vi "Filter_Table_Test.vi"() -> ()   [LabVIEW 2025, in "Table_Filtering.lvlib"]
uses:
  Table_Filtering.lvlib
  <vilib>/Utility/miscctls.llb/LVRowAndColumnUnsignedTypeDef.ctl
panel:
  out "Error Out":errorcluster
  in  "Filter String":string="Protocol == UDP AND Length > 0.7 OR Source == 192.168.1.1 AND Hex_Data < 20"
  in  "Sort by":u16(ring) items=["Packet_Number", "Timestamp", "Source", "Destination", "Protocol", "Length", "Data", "Hex_Data"]
  in  "Headers and Types":string[][](array[string])=[["Packet_Number", "Timestamp", "Source", "Destination", "Protocol", "Length", "Data", "Hex_Data"], ["NUM", "STR", "STR", "STR", "STR", "NUM", "STR", "HEX"]]
  in  "Pause":bool
  out "Table Control":string[][](table)
  in  "stop":bool
  in  "Visible Columns":bool[](array[boolean])=[TRUE, TRUE, TRUE, TRUE, TRUE, TRUE, TRUE, TRUE]
  # "The filter expression uses the following syntax:\n\nSets of three arguments separated by logical operators.\nSpaces are used to separate keywords.\nEach set of three arguments follows the pattern: Field, Operator, Value.\nExample: \nProtocol == UDP AND Length > 0.7 OR Source == 192.168.1.1\n\nInvalid inputs include:\n\nStandalone logical operators (e.g., AND, OR)\nTerms by themselves\nArgument sets not equal to three in length\nParentheses\nIf an invalid filter is entered, a warning will be generated."
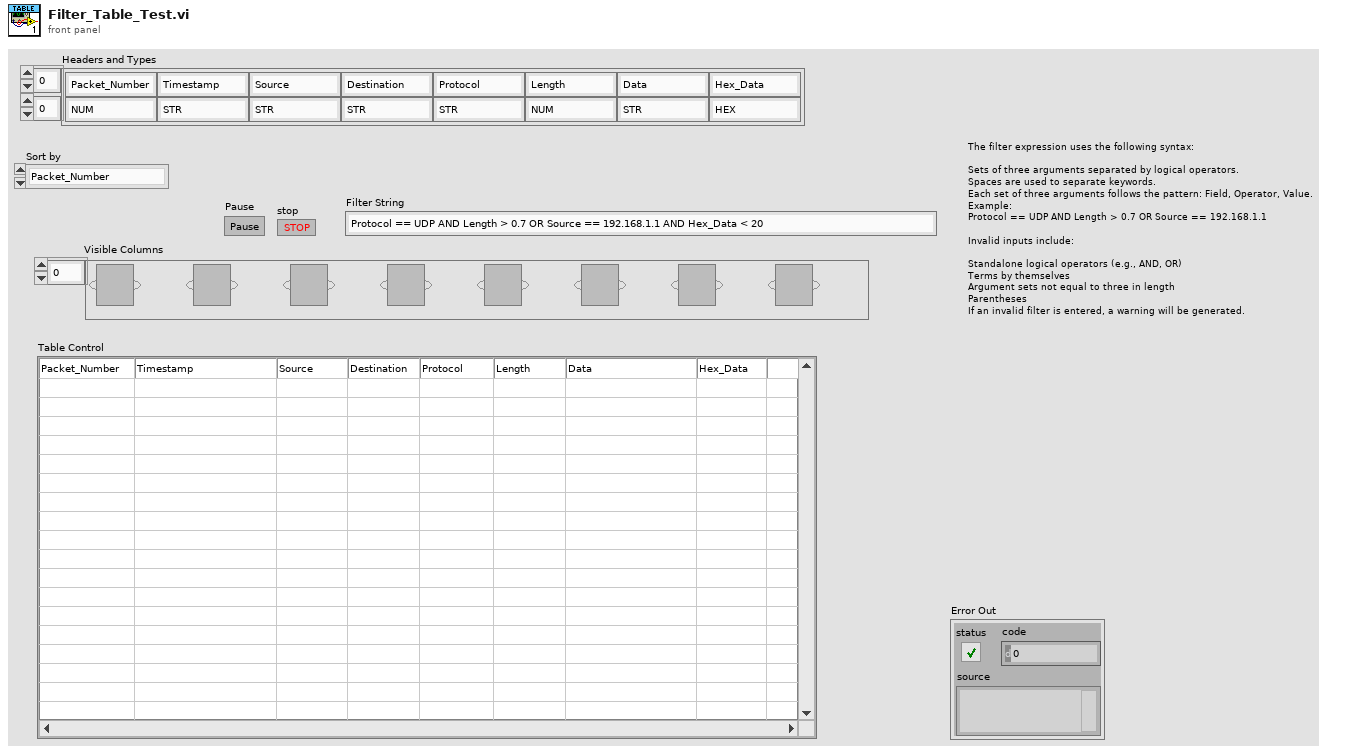
[diagram p1: front panel]
types:
  T1 = typedef "LVRowAndColumnUnsignedTypeDef.ctl" = cluster{"Row":u32, "Column":u32}
  T2 = cluster{"FIELD":string, "OPERATOR":string, "VALUE":string}[]
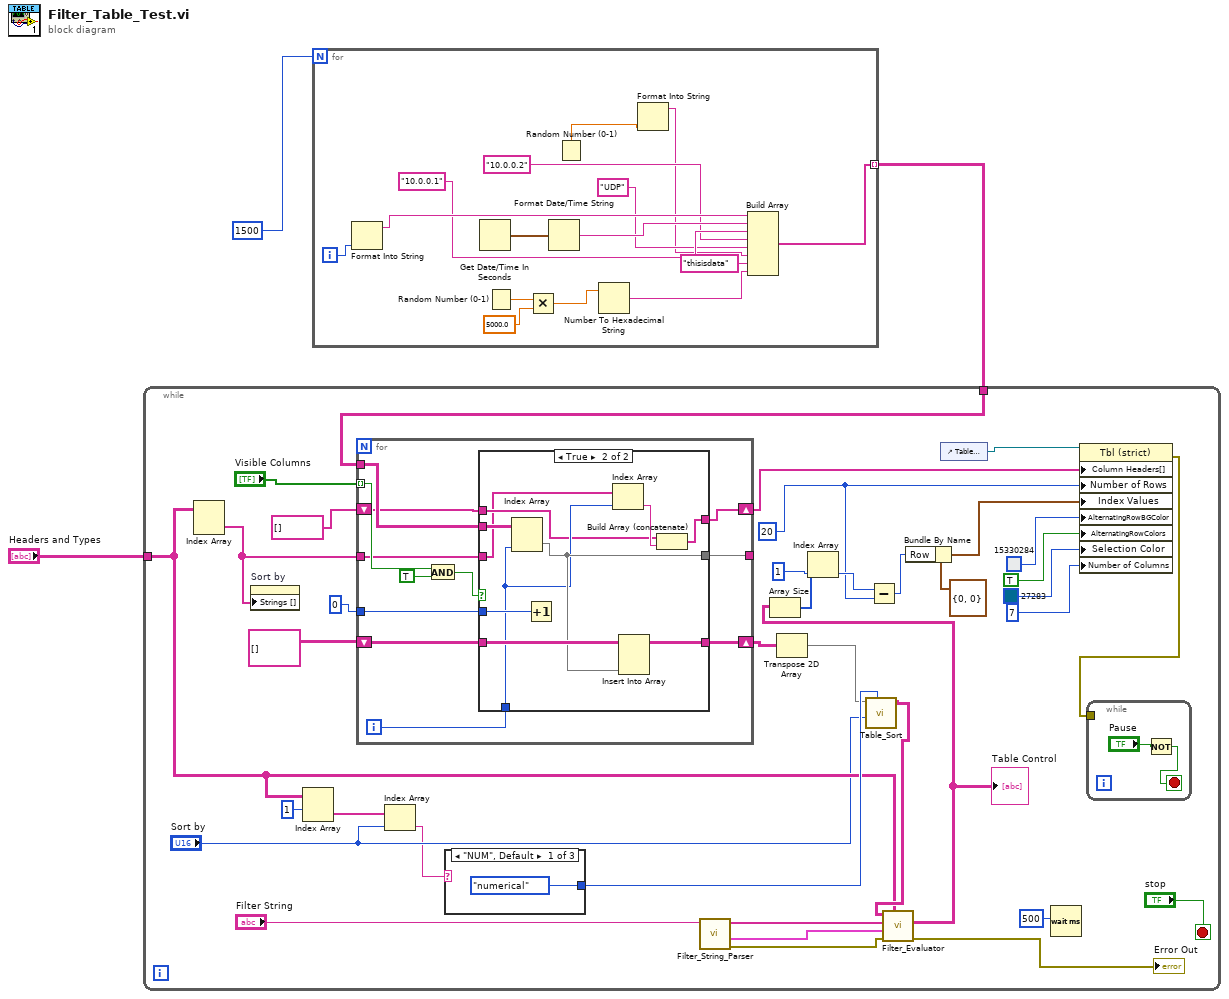
[diagram p0: block diagram]
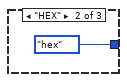
[diagram p2: hidden frame]
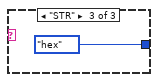
[diagram p3: hidden frame]
diagram:
  n1 = for {
    N: 1500 ("Numeric") -> [_]
    tunnel: [w18] -> w2 mode=indexing
    i -> [w17]
    n2 = Format Into String(w17) -> (resulting string=w16:string)  [unwired: 3 in, 1 out]
    n3 = Get Date/Time In Seconds() -> (seconds since 1Jan1904=w15:timestamp)
    n4 = Random Number (0-1)() -> (number: 0 to 1=w7:dbl)
    n5 = Multiply(x=w7, y=5000.0) -> (x*y=w5:dbl)
    n6 = Format Date/Time String(seconds (now)=w15) -> (date/time string=w14:string)  [unwired: 2 in]
    n7 = Random Number (0-1)() -> (number: 0 to 1=w10:dbl)
    n8 = Number To Hexadecimal String(2:w5) -> (0:w4:string)  [unwired: 1 in]
    n9 = Format Into String(w10) -> (resulting string=w9:string)  [unwired: 3 in, 1 out]
    n10 = Build Array(w16, w14, "10.0.0.1", "10.0.0.2", "UDP", w9, "thisisdata" ("element"), w4) -> (w18:string[])
  }
  n11 = while {
    tunnel: w2 -> [w55]
    tunnel: "Headers and Types" -> [w24]
    stop <- "stop" stop-if-true
    w46 = u32 20 ("Number of Rows")
    n12 = Index Array(array=w24) -> (element=w25:string[])  [unwired: 2 in]
    n13 = property on="Sort by" class="Ring (strict)"("Strings []"=w25) -> ()  [unwired: 2 in, 2 out]
    n14 = Index Array(array=w24, index (row)=1) -> (element=w22:string[])  [unwired: 1 in]
    n15 = for {
      tunnel: "Visible Columns" -> [w70] mode=indexing
      tunnel: w55 -> [w72]
      tunnel: [w67] -> _
      shift-right: [w66] -> w50
      shift-left: string[][] [] ("array") -> [w68]
      tunnel: 0 -> [w64]
      shift-right: [w62] -> w52
      shift-left: string[] [] -> [w63]
      tunnel: w25 -> [w61]
      i -> [w71]
      n16 = And(x=w70, y=TRUE) -> (x .and. y?=w65:bool)
      n17 = case shown="True" w65 {
        tunnel: w72 -> [_ w84]
        tunnel: w71 -> [_ w79]
        tunnel: w68 -> [w74 w83]
        tunnel: [_ w82] -> w67
        tunnel: [w74 w81] -> w66
        tunnel: w64 -> [_ w80]
        tunnel: [w73 w78] -> w62
        tunnel: w63 -> [w73 w76]
        tunnel: w61 -> [_ w75]
        frame False {
        }
        frame True {
          n18 = Index Array(array=w84, index (col)=w79) -> (element=w82:string[])  [unwired: 1 in]
          n19 = Increment(x=w80) -> ()  [unwired: 1 out]
          n20 = Index Array(array=w75, index=w79) -> (element=w77:string)
          n21 = Insert Into Array(array=w83, new element=w82) -> (w81:string[][])  [unwired: 2 in]
          n22 = Build Array (concatenate)(w76, w77) -> (w78:string[])
        }
      }
    }
    n23 = Index Array(array=w22, index="Sort by") -> (element=w20:string)
    n24 = case shown="\"NUM\", Default" w20 {
      tunnel: [enum16{"numerical", "hex", "string"}."numerical" ("Sort Type") enum16{"numerical", "hex", "string"}."hex" ("Sort Type") enum16{"numerical", "hex", "string"}."hex" ("Sort Type")] -> w28
      frame "NUM", Default {
      }
      frame "HEX" {
      }
      frame "STR" {
      }
    }
    n25 = call "Filter_String_Parser.vi"("Filter String"="Filter String") -> ("error constant"=w27:errorcluster, "Comparators"=w32:T2, "Boolean Connectors"=w31:string[])  [unwired: 8 in]
    n26 = Transpose 2D Array(2D array=w50) -> (transposed array=w19:string[][])
    n27 = call "Table_Sort.vi"("Sort Type"=w28, "Sort by"="Sort by", "Unsorted Data"=w19) -> ("Sorted data"=w29:string[][])  [unwired: 8 in]
    n28 = call "Filter_Evaluator.vi"("Headers and Types"=w24, "Error"=w27, "Comparators"=w32, "Boolean Connectors"=w31, "Prefiltered Data"=w29) -> ("Error Out"=→"Error Out":errorcluster, "Filtered Array"=w30:string[][])  [unwired: 4 in, 1 out]
    "Table Control" <- w30
    n29 = Array Size(array=w30) -> (size(s)=w49:i32[])
    n30 = Index Array(array=w49, index=1) -> (element=w47:i32)
    n31 = Subtract(x=w47, y=w46) -> (x-y=w45:u32)
    n32 = Bundle By Name(cluster=T1 {"Row"=0, "Column"=0} ("Index Values"), "Row"=w45) -> (w44:T1)
    n33 = control-ref of="Table Control"() -> (w36:refnum<vi>)
    n34 = Wait (ms)(milliseconds to wait=u32 500) -> ()  [unwired: 1 out]
    n35 = property on="Property Node" class="Tbl (strict)"(reference=w36, "Column Headers[]"=w52, "Number of Rows"=w46, "Index Values"=w44, "AlternatingRowBGColor"=u32 15330284 ("Alternate Row Background Color"), "AlternatingRowColors"=TRUE ("Alternating Row Colors"), "Selection Color"=u32 27283, "Number of Columns"=u32 7) -> (error out=w37:errorcluster)  [unwired: 1 in, 1 out]
    n36 = while {
      tunnel: w37 -> [_]
      stop <- w59 stop-if-true
      n37 = Not(x="Pause") -> (.not. x?=w59:bool)
    }
  }
